vi "niRFSG IVI Error Converter.vi"(8 "error in":errorcluster {"code" format="%.0x"}, 9 "instrument handle":u32, 10 "IVI error code":i32 format="%.0x", 11 "path to VI":path) -> (0 "error out":errorcluster {"code" format="%.0x"})   [LabVIEW 2014]
doc: "This VI converts error codes from IVI instrument drivers to standard LabVIEW error codes. If an error is detected the VI builds the appropriate error cluster that is readable by one of the error handlers supplied with LabVIEW."
uses:
  niRFSG.dll
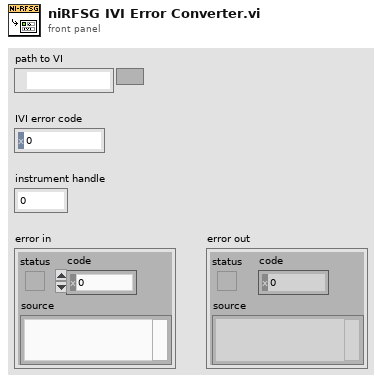
[diagram p1: front panel]
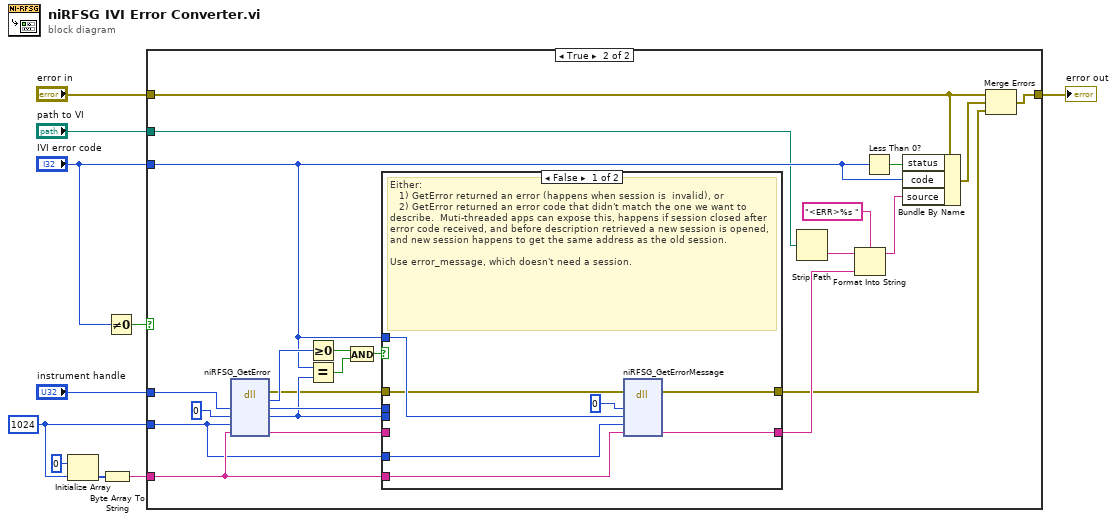
[diagram p0: block diagram]
diagram:
  w1 = 1024 ("dimension size")
  n1 = Initialize Array(u8 0, w1) -> (w4:u8[])
  n2 = Byte Array To String(unsigned byte array=w4) -> (string=w2:string)
  n3 = Not Equal To 0?(x="IVI error code") -> (x != 0?=w8:bool)
  n4 = case shown="True" w8 {
    tunnel: [w11 w28] -> w7
    tunnel: "IVI error code" -> [_ w21]
    tunnel: "error in" -> [w11 w27]
    tunnel: "instrument handle" -> [_ w15]
    tunnel: "path to VI" -> [_ w14]
    tunnel: w2 -> [_ w13]
    tunnel: w1 -> [_ w12]
    frame False {
    }
    frame True {
      n5 = dll-call lib="niRFSG**.*" fn="niRFSG_GetError" label="GetError"("vi"=w15, "errorCode"=0, "bufferSize"=w12, "description"=w13) -> (error out=w17:errorcluster, w26:i32, "vi"=w33:u32, "errorCode"=w20:i32, "description"=w18:string)  [unwired: 4 in, 1 out]
      n6 = Greater Or Equal To 0?(x=w26) -> (x >= 0?=w23:bool)
      n7 = Equal?(x=w21, y=w20) -> (x = y?=w22:bool)
      n8 = And(x=w23, y=w22) -> (x .and. y?=w24:bool)
      n9 = case shown="False" w24 {
        tunnel: w33 -> [_ _]
        tunnel: w20 -> [_ _]
        tunnel: [w40 w43] -> w25
        tunnel: w21 -> [w41 _]
        tunnel: w18 -> [_ w43]
        tunnel: w17 -> [w38 w42]
        tunnel: [w37 w42] -> w16
        tunnel: w13 -> [w36 _]
        tunnel: w12 -> [w35 _]
        frame False {
          # "Either:\n   1) GetError returned an error (happens when session is  invalid), or\n   2) GetError returned an error code that didn't match the one we want to describe.  Muti-threaded apps can expose this, happens if session closed after error code received, and before description retrieved a new session is opened, and new session happens to get the same address as the old session.\n\nUse error_message, which doesn't need a session."
          n10 = dll-call lib="niRFSG**.*" fn="niRFSG_GetErrorMessage" label="GetErrorMessage"(error in=w38, "instrumentHandle"=0, "errorCode"=w41, "errorDescriptionBufferSize"=w35, "errorDescription"=w36) -> (error out=w37:errorcluster, "errorDescription"=w40:string)  [unwired: 6 in, 1 out]
        }
        frame True {
          # "Call to GetError was successful, and it returned a description that matched the error code we passed."
        }
      }
      n11 = Strip Path(path=w14) -> (name=w30:string)  [unwired: 1 out]
      n12 = Format Into String(format string="<ERR>%s ", initial string=w30, w25) -> (resulting string=w31:string)  [unwired: 1 in, 1 out]
      n13 = Less Than 0?(x=w21) -> (x < 0?=w34:bool)
      n14 = Bundle By Name(cluster=w27, "status"=w34, "code"=w21, "source"=w31) -> (w29:errorcluster)
      n15 = Merge Errors(w27, w29, w16) -> (w28:errorcluster)
    }
  }
  "error out" <- w7
